vi "CC Observation Queue GUI.vi"() -> ()   [LabVIEW 2024]
uses:
  Subsystems/SS cluster Script Status Queue.ctl
  typedefs/CC cluster Observation.ctl
  CC enum Observation Status.ctl
  Telescope/CC cluster Telescope Offsets.ctl
  typedefs/CC cluster Observation Dither Options.ctl
  typedefs/CC enum Dither Selection.ctl
  Subsystems/SS typedef cluster Instrument Command Queue Data.ctl
  CC cluster Script State.ctl
  CC cluster Observation Settings.ctl
  CC cluster Air Mass Data.ctl
  Logging/CC enum Current Values Action.ctl
  typedefs/CC cluster Script.ctl
  typedefs/CC Script Step.ctl
  typedefs/CC enum Script Action.ctl
  Scripts/CC Rd Wr Script Action.ctl
  hk-channel-class/hk-channel-class/HK Table/HK Table.lvclass
panel:
  in  "Open Plots":bool
  in  "Air Mass Tool":bool
  out "Row":i32 caption="Next"
  in  "queue idle":string="TELESCOPE IDLE"
  in  "clean table":bool
  in  "Auto Step":bool
  in  "Stop":bool
  out "Queue Running":i16(slide) scale=-1.0..70.0
  in  "Pause Q":bool
  in  "Run Queue":bool
  in  "Close":bool
  out "Queue":i32(listbox)
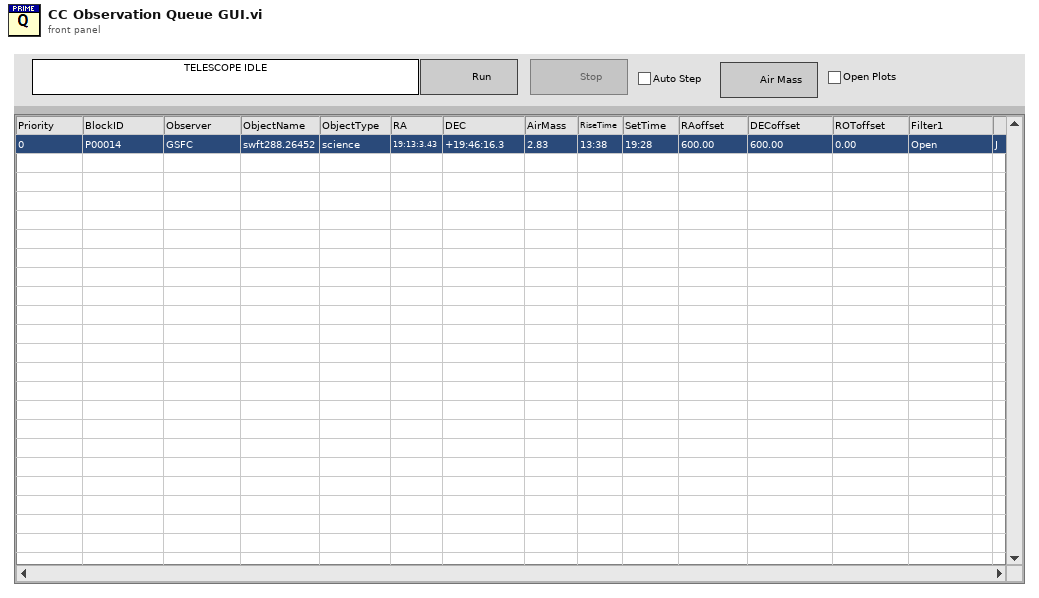
[diagram p1: front panel]
types:
  T1 = typedef "CC cluster Observation.ctl" = cluster{"Priority":i32, "ID":string, "Observer":string, "Obj Name":string, "Obj Type":string, "RA and DEC String":cluster{"RA":string, "DEC":string}, "Filter Wheel 1":string, "Filter Wheel 2":string, "Integration Time":dbl, "Observation Status":T2, "Offsets":T3, "Images":i32, "Dither Options":T4, "Comment 1":string, "Comment 2":string}
  T2 = typedef "CC enum Observation Status.ctl" = enum16{"Ready", "Running", "Done", "Error"}
  T3 = typedef "CC cluster Telescope Offsets.ctl" = cluster{"RA":dbl, "DEC":dbl, "ROT":dbl}
  T4 = typedef "CC cluster Observation Dither Options.ctl" = cluster{"Dither":T5, "Dither Radius":dbl, "Dither Points":i32, "Dither Phase":dbl}
  T5 = typedef "CC enum Dither Selection.ctl" = enum16{"None", "Circle", "Random"}
  T6 = typedef "CC cluster Script State.ctl" = cluster{"Image Count":i32, "Step":i32, "Dither Idx":i32, "Dither Total":i32, "Running":bool, "State":u16}
  T7 = typedef "CC cluster Observation Settings.ctl" = cluster{"Air Mass Program Path":path}
  T8 = typedef "CC cluster Air Mass Data.ctl" = cluster{"BlockID":string, "Air Mass":string, "Rise Time":string, "Set Time":string}
  T9 = cluster{"state":refnum<user-event>, "Obs Queue":refnum<queue>, "Observation List":T1[], "Data":variant, "Obs State":enum16{"Idle", "Running", "Paused"}, "Row":i32, "Script Q":refnum<queue>, "Expected Images":i32, "Script Status":T6, "Prev Status":T6, "script name":string, "Observation Settings":T7, "BlockIDs":string[], "Airmass Idx":i32, "Air Mass":T8[]}
  T10 = typedef "CC enum Current Values Action.ctl" = enum16{"Init", "Write Item", "Write Array", "Read Item", "Read Array", "Read All", "Add Channels", "New File", "Add Message", "Get Current Values", "Close"}
  T11 = enum8{"Enabled", "Disabled", "Disabled and Grayed Out"}
  T12 = typedef "SS typedef cluster Instrument Command Queue Data.ctl" = cluster{"Cmd":string, "Parameters":variant}
  T13 = typedef "CC Rd Wr Script Action.ctl" = enum16{"Read", "Write", "List", "Delete"}
  T14 = typedef "CC cluster Script.ctl" = cluster{"Name":string, "Script":T15[]}
  T15 = typedef "CC Script Step.ctl" = cluster{"Action":T16, "Data":variant}
  T16 = typedef "CC enum Script Action.ctl" = enum16{"Noop", "Define Object", "Define Exposure", "Define Dithering", "Acquire Images", "Set Filter Wheel", "Telescope Home", "Telescope Move", "Telescope RA DEC", "Focus Move Relative", "Focus Move Absolute", "Focus Set Home", "Macro", "Pause", "Ask User", "Define Random Dither"}
  T17 = typedef "SS cluster Script Status Queue.ctl" = cluster{"Msg":string, "Data":variant}
  T18 = typedef "CC cluster Script Panel Defaults.ctl" = cluster{"Script Name":string, "Script Path":path}
  T19 = typedef "LVPoint32TypeDef.ctl" = cluster{"Horizontal":i32, "Vertical":i32}
  T20 = typedef "LVRowAndColumnTypeDef.ctl" = cluster{"Row":i32, "Column":i32}
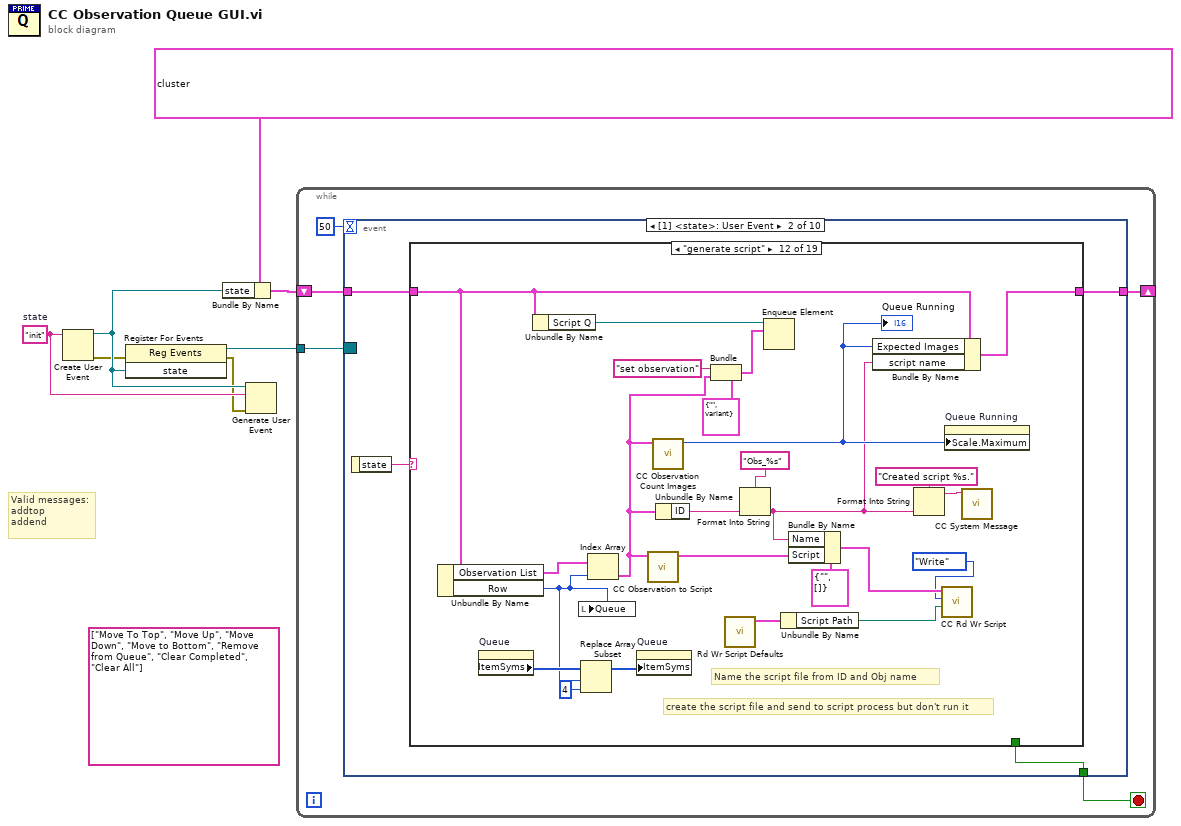
[diagram p0: block diagram]
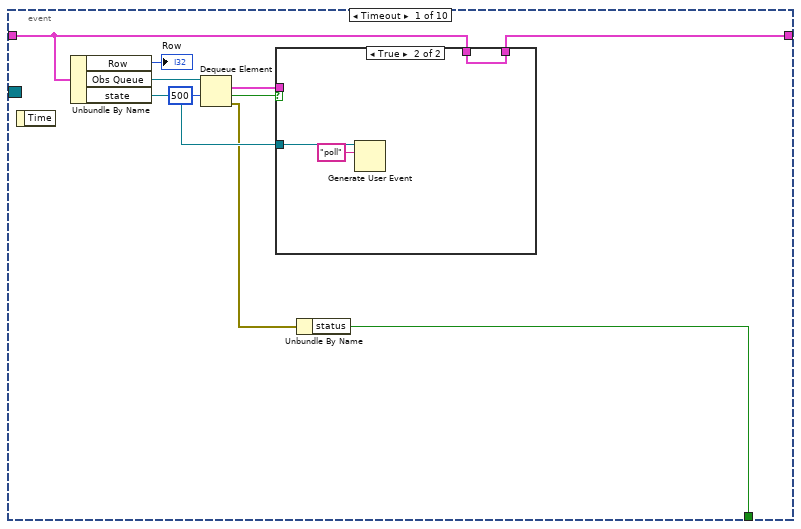
[diagram p2: hidden frame]
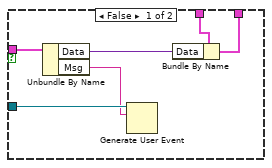
[diagram p3: hidden frame]
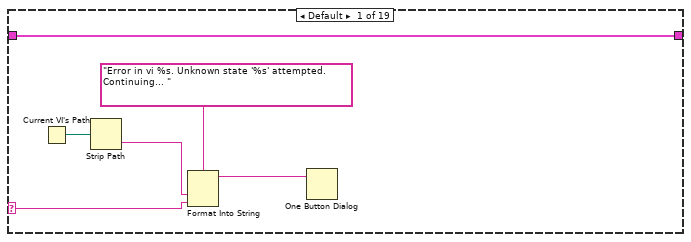
[diagram p4: hidden frame]
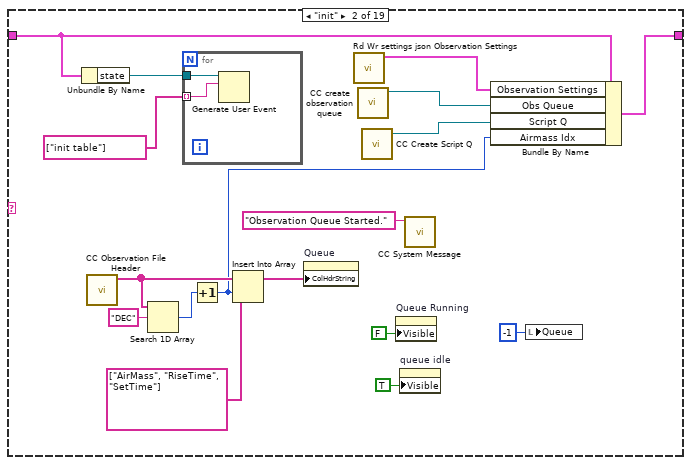
[diagram p5: hidden frame]
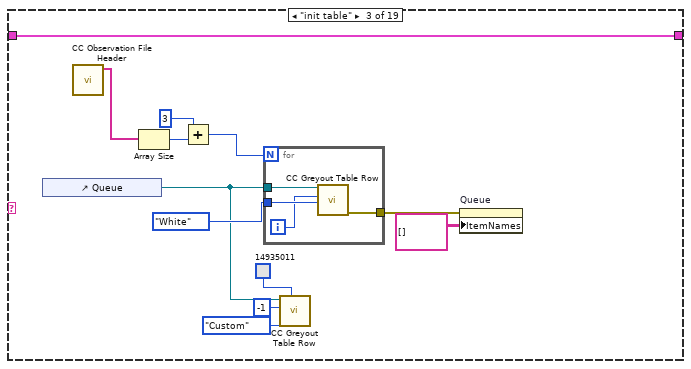
[diagram p6: hidden frame]
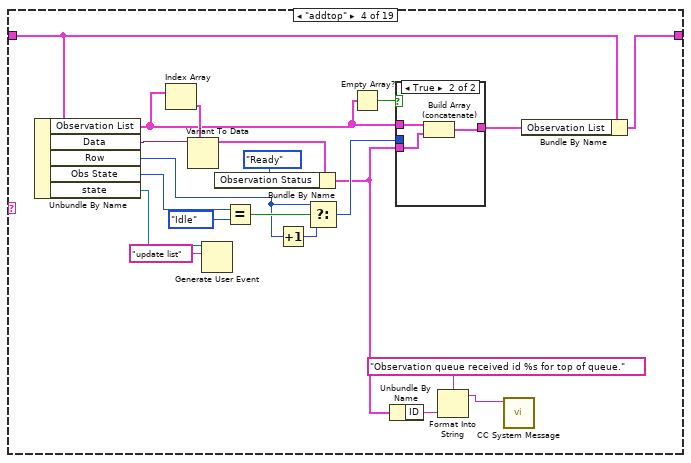
[diagram p7: hidden frame]
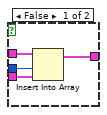
[diagram p8: hidden frame]
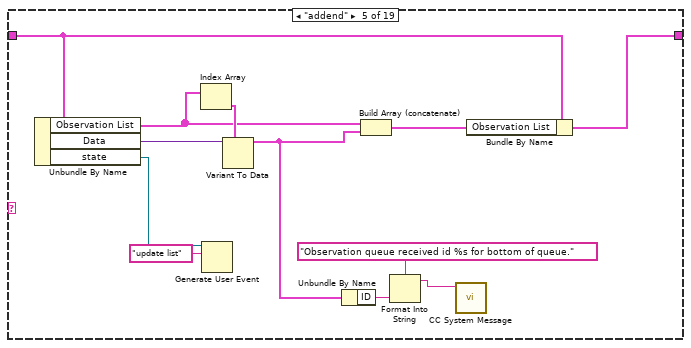
[diagram p9: hidden frame]
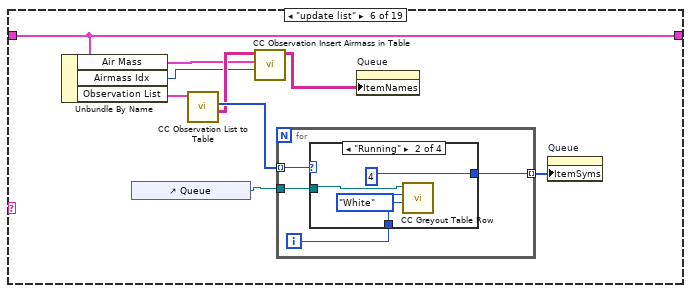
[diagram p10: hidden frame]
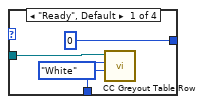
[diagram p11: hidden frame]
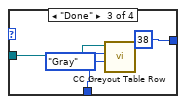
[diagram p12: hidden frame]
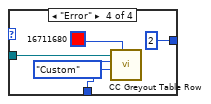
[diagram p13: hidden frame]
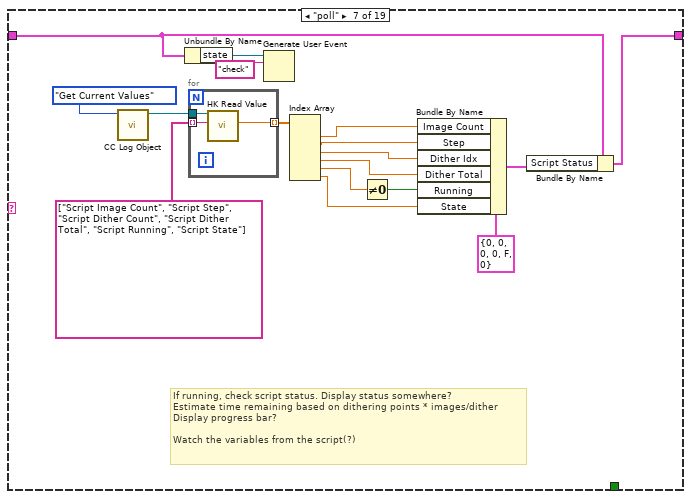
[diagram p14: hidden frame]
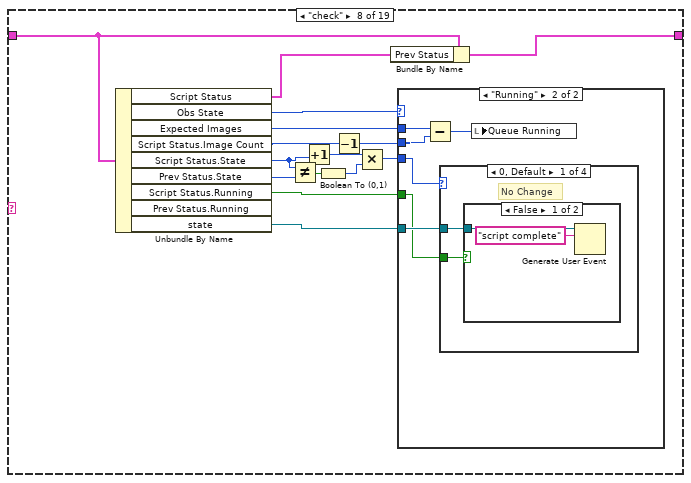
[diagram p15: hidden frame]
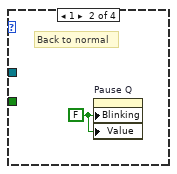
[diagram p18: hidden frame]
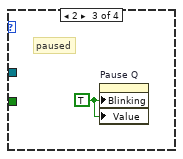
[diagram p19: hidden frame]
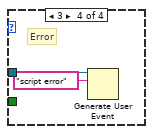
[diagram p20: hidden frame]
diagram:
  (unwired) string[] ["Move To Top", "Move Up", "Move Down", "Move to Bottom", "Remove from Queue", "Clear Completed", "Clear All"]
  w3 = "init"  # state
  # "Valid messages:\naddtop\naddend"
  n1 = Create User Event(user event datatype=w3) -> (user event=w5:refnum<user-event>, error out=w1:errorcluster)  [unwired: 1 in]
  n2 = register-events(error in=w1, w5) -> (reference out=w4:refnum<event-registration>, error out=w2:errorcluster)  [unwired: 1 in]
  n3 = Bundle By Name(cluster=T9 {"state"=refnum, "Obs Queue"=refnum, "Observation List"=[], "Data"=variant, "Obs State"=enum."Idle", "Row"=0, "Script Q"=refnum, "Expected Images"=0, "Script Status"={"Image Count"=0, "Step"=0, "Dither Idx"=0, "Dither Total"=0, "Running"=FALSE, "State"=0}, "Prev Status"={"Image Count"=0, "Step"=0, "Dither Idx"=0, "Dither Total"=0, "Running"=FALSE, "State"=0}, "script name"="", "Observation Settings"={"Air Mass Program Path"=path ""}, "BlockIDs"=["P0102", "P00002", "P00003", "P00004", "P00005", "P00006"], "Airmass Idx"=0, "Air Mass"=[{"BlockID"="", "Air Mass"="", "Rise Time"="06:16", "Set Time"="13:33"}, {"BlockID"="", "Air Mass"="", "Rise Time"="06:16", "Set Time"="13:33"}, {"BlockID"="", "Air Mass"="", "Rise Time"="06:16", "Set Time"="13:33"}, {"BlockID"="", "Air Mass"="", "Rise Time"="06:16", "Set Time"="13:33"}, {"BlockID"="", "Air Mass"="", "Rise Time"="06:16", "Set Time"="13:33"}, {"BlockID"="", "Air Mass"="", "Rise Time"="06:16", "Set Time"="13:33"}]}, "state"=w5) -> (w6:T9)
  n4 = Generate User Event(user event=w5, event data cluster=w3, error in=w2) -> ()  [unwired: 1 in, 2 out]
  n5 = while {
    tunnel: w4 -> [w12]
    shift-right: [w10] -> _
    shift-left: w6 -> [w11]
    stop <- w9 stop-if-true
    n6 = event shown="[1] <state>: User Event" {
      selector: w12 -> [_ _ _ _ _ _ _ _ _ _]
      dyn-events: _ -> [_ _ _ _ _ _ _ _ _ _]
      timeout: 50 -> [_ _ _ _ _ _ _ _ _ _]
      tunnel: w11 -> [w17 w34 w369 w401 w470 w543 w549 w554 w558 w560]
      tunnel: [w18 w33 w370 w401 w471 w543 w549 w554 w558 w560] -> w10
      tunnel: [w14 w32 _ _ _ _ _ _ _ "Close"] -> w9
      event Timeout {
        n7 = event-data() -> ()  [unwired: 1 in, 1 out]
        n8 = Unbundle By Name(w17) -> ("Row"=→"Row":i32, "Obs Queue"=w22:refnum<queue>, "state"=w19:refnum<user-event>)
        n9 = Dequeue Element(queue=w22, timeout in ms (-1)=500) -> (element=w20:T17, timed out?=w21:bool, error out=w15:errorcluster)  [unwired: 1 in, 1 out]
        n10 = case shown="True" w21 {
          tunnel: w20 -> [w28 _]
          tunnel: w19 -> [w27 w30]
          tunnel: w17 -> [w25 w31]
          tunnel: [w23 w31] -> w18
          frame False {
            n11 = Unbundle By Name(w28) -> ("Data"=w24:variant, "Msg"=w26:string)
            n12 = Generate User Event(user event=w27, event data cluster=w26) -> ()  [unwired: 2 in, 2 out]
            n13 = Bundle By Name(cluster=w25, "Data"=w24) -> (w23:T9)
          }
          frame True {
            n14 = Generate User Event(user event=w30, event data cluster="poll" ("event data")) -> ()  [unwired: 2 in, 2 out]
          }
        }
        n15 = Unbundle By Name(w15) -> ("status"=w14:bool)
      }
      event User Event {
        n16 = event-data() -> ("state"=w35:string)  [unwired: 1 in]
        n17 = case shown="\"generate script\"" w35 {
          selector: w35 -> [w40 _ _ _ _ _ _ _ _ _ _ _ _ _ _ _ _ _ _]
          tunnel: w34 -> [w36 w54 w72 w93 w111 w125 w150 w168 w202 w228 w232 w262 w285 w306 w326 w335 w351 w361 w366]
          tunnel: [w36 w57 w72 w94 w112 w125 w151 w169 w203 w229 w233 w273 w286 w307 w326 w336 w352 w361 w366] -> w33
          tunnel: [_ _ _ _ _ _ _ _ _ _ _ _ _ _ _ _ _ _ TRUE] -> w32
          frame Default {
            n18 = Current VI's Path() -> (path=w39:path)
            n19 = Strip Path(path=w39) -> (name=w38:string)  [unwired: 1 out]
            n20 = Format Into String(format string="Error in vi %s. Unknown state '%s' attempted. Continuing... ", w38, w40) -> (resulting string=w37:string)  [unwired: 2 in, 1 out]
            n21 = One Button Dialog(message=w37) -> ()  [unwired: 1 in, 1 out]
          }
          frame "init" {
            n22 = Unbundle By Name(w54) -> ("state"=w53:refnum<user-event>)
            n23 = call "CC Observation File Header.vi"() -> ("Header"=w47:string[])  [unwired: 10 in, 1 out]
            n24 = Search 1D Array(1D array=w47, element="DEC") -> (index of element=w44:i32)  [unwired: 1 in]
            n25 = for {
              tunnel: w53 -> [w60]
              tunnel: string[] ["init table"] -> [w59] mode=indexing
              n26 = Generate User Event(user event=w60, event data cluster=w59) -> ()  [unwired: 2 in, 2 out]
            }
            n27 = Increment(x=w44) -> (x+1=w42:i32)
            n28 = Insert Into Array(array=w47, index=w42, new element=string[] ["AirMass", "RiseTime", "SetTime"]) -> (w45:string[])
            n29 = property on="Queue" class="MCListbox (strict)"("ColHdrString"=w45) -> ()  [unwired: 2 in, 2 out]
            n30 = call "Rd Wr settings json Observation Settings.vi"() -> ("Observation Settings"=w48:T7)  [unwired: 10 in, 1 out]
            n31 = call "CC create observation queue.vi"() -> ("Observation Queue"=w58:refnum<queue>)  [unwired: 10 in, 1 out]
            n32 = call "CC Create Script Q.vi"() -> ("Script Q"=w56:refnum<queue>)  [unwired: 10 in, 1 out]
            n33 = property on="Queue Running" class="Slide (strict)"("Visible"=FALSE) -> ()  [unwired: 2 in, 2 out]
            n34 = property on="queue idle" class="Str"("Visible"=TRUE) -> ()  [unwired: 2 in, 2 out]
            n35 = call "CC System Message.vi"("Message"="Observation Queue Started.") -> ()  [unwired: 10 in, 1 out]
            n36 = Bundle By Name(cluster=w54, "Observation Settings"=w48, "Obs Queue"=w58, "Script Q"=w56, "Airmass Idx"=w42) -> (w57:T9)
            n37 = local write "Queue"(-1 ("Queue")) -> ()
          }
          frame "init table" {
            n38 = control-ref of="Queue"() -> (w68:refnum<vi>)
            n39 = call "CC Observation File Header.vi"() -> ("Header"=w64:string[])  [unwired: 10 in, 1 out]
            n40 = Array Size(array=w64) -> (size(s)=w63:i32)
            n41 = Add(x=3, y=w63) -> (x+y=w62:i32)
            n42 = for {
              N: w62 -> [_]
              tunnel: w68 -> [w76]
              tunnel: [w75] -> w71
              tunnel: enum16{"White", "Gray", "Custom"}."White" ("Color") -> [w74]
              i -> [w73]
              n43 = call "CC Greyout Table Row.vi"("Color"=w74, "Row"=w73, "Queue ref"=w76) -> ("error out"=w75:errorcluster)  [unwired: 8 in]
            }
            n44 = call "CC Greyout Table Row.vi"("Color Box"=u32 14935011, "Color"=enum16{"White", "Gray", "Custom"}."Custom", "Row"=-1, "Queue ref"=w68) -> ()  [unwired: 7 in, 1 out]
            n45 = property on="Queue" class="MCListbox (strict)"(error in=w71, "ItemNames"=string[][] [] ("Item Names")) -> ()  [unwired: 1 in, 2 out]
          }
          frame "addtop" {
            n46 = Unbundle By Name(w93) -> ("Observation List"=w82:T1[], "Data"=w97:variant, "Row"=w77:i32, "Obs State"=w92:enum16{"Idle", "Running", "Paused"}, "state"=w87:refnum<user-event>)
            n47 = Index Array(array=w82) -> (element=w96:T1)  [unwired: 1 in]
            n48 = Variant To Data(type=w96, Variant=w97) -> (data=w81:T1)  [unwired: 1 in, 1 out]
            n49 = Generate User Event(user event=w87, event data cluster="update list" ("event data")) -> ()  [unwired: 2 in, 2 out]
            n50 = Bundle By Name(cluster=w81, "Observation Status"=CC_enum_Observation_Status."Ready") -> (w79:T1)
            n51 = Equal?(x=w92, y=enum16{"Idle", "Running", "Paused"}."Idle") -> (x = y?=w90:bool)
            n52 = Increment(x=w77) -> (x+1=w88:i32)
            n53 = Select(t=w77, s=w90, f=w88) -> (s? t:f=w89:i32)
            n54 = Empty Array?(array=w82) -> (empty?=w78:bool)
            n55 = Unbundle By Name(w79) -> ("ID"=w84:string)
            n56 = case shown="True" w78 {
              tunnel: [w101 w102] -> w95
              tunnel: w89 -> [w100 _]
              tunnel: w82 -> [w99 w104]
              tunnel: w79 -> [w98 w103]
              frame False {
                n57 = Insert Into Array(array=w99, index=w100, new element=w98) -> (w101:T1[])
              }
              frame True {
                n58 = Build Array (concatenate)(w104, w103) -> (w102:T1[])
              }
            }
            n59 = Format Into String(format string="Observation queue received id %s for top of queue.", w84) -> (resulting string=w83:string)  [unwired: 2 in, 1 out]
            n60 = call "CC System Message.vi"("Message"=w83) -> ()  [unwired: 10 in, 1 out]
            n61 = Bundle By Name(cluster=w93, "Observation List"=w95) -> (w94:T9)
          }
          frame "addend" {
            n62 = Unbundle By Name(w111) -> ("Observation List"=w114:T1[], "Data"=w116:variant, "state"=w110:refnum<user-event>)
            n63 = Index Array(array=w114) -> (element=w115:T1)  [unwired: 1 in]
            n64 = Generate User Event(user event=w110, event data cluster="update list" ("event data")) -> ()  [unwired: 2 in, 2 out]
            n65 = Variant To Data(type=w115, Variant=w116) -> (data=w105:T1)  [unwired: 1 in, 1 out]
            n66 = Unbundle By Name(w105) -> ("ID"=w107:string)
            n67 = Build Array (concatenate)(w114, w105) -> (w113:T1[])
            n68 = Format Into String(format string="Observation queue received id %s for bottom of queue.", w107) -> (resulting string=w106:string)  [unwired: 2 in, 1 out]
            n69 = call "CC System Message.vi"("Message"=w106) -> ()  [unwired: 10 in, 1 out]
            n70 = Bundle By Name(cluster=w111, "Observation List"=w113) -> (w112:T9)
          }
          frame "update list" {
            n71 = Unbundle By Name(w125) -> ("Air Mass"=w119:T8[], "Airmass Idx"=w118:i32, "Observation List"=w124:T1[])
            n72 = control-ref of="Queue"() -> (w121:refnum<vi>)
            n73 = call "CC Observation List to Table.vi"("Observation List"=w124) -> ("Screen Ready Table"=w120:string[][], "Status"=w123:T2[])  [unwired: 7 in, 2 out]
            n74 = call "CC Observation Insert Airmass in Table.vi"("Airmass Idx"=w118, "Air Mass"=w119, "Table"=w120) -> ("Table out"=w117:string[][])  [unwired: 8 in]
            n75 = for {
              tunnel: w123 -> [w129] mode=indexing
              tunnel: [w128] -> w122 mode=indexing
              tunnel: w121 -> [w126]
              i -> [w127]
              n76 = case shown="\"Running\"" w129 {
                tunnel: [0 4 ("new element/subarray") 38 ("new element/subarray") 2 ("new element/subarray")] -> w128
                tunnel: w127 -> [w132 w137 w140 w143]
                tunnel: w126 -> [w130 w136 w139 w145]
                frame "Ready", Default {
                  n77 = call "CC Greyout Table Row.vi"("Color"=enum16{"White", "Gray", "Custom"}."White", "Row"=w132, "Queue ref"=w130) -> ()  [unwired: 8 in, 1 out]
                }
                frame "Running" {
                  n78 = call "CC Greyout Table Row.vi"("Color"=enum16{"White", "Gray", "Custom"}."White", "Row"=w137, "Queue ref"=w136) -> ()  [unwired: 8 in, 1 out]
                }
                frame "Done" {
                  n79 = call "CC Greyout Table Row.vi"("Color"=enum16{"White", "Gray", "Custom"}."Gray", "Row"=w140, "Queue ref"=w139) -> ()  [unwired: 8 in, 1 out]
                }
                frame "Error" {
                  n80 = call "CC Greyout Table Row.vi"("Color Box"=u32 16711680, "Color"=enum16{"White", "Gray", "Custom"}."Custom", "Row"=w143, "Queue ref"=w145) -> ()  [unwired: 7 in, 1 out]
                }
              }
            }
            n81 = property on="Queue" class="MCListbox (strict)"("ItemNames"=w117) -> ()  [unwired: 2 in, 2 out]
            n82 = property on="Queue" class="MCListbox (strict)"("ItemSyms"=w122) -> ()  [unwired: 2 in, 2 out]
          }
          frame "poll" {
            # "If running, check script status. Display status somewhere?\nEstimate time remaining based on dithering points * images/dither\nDisplay progress bar?\n\nWatch the variables from the script(?)"
            n83 = call "CC Log Object.vi"("Action"=CC_enum_Current_Values_Action."Get Current Values") -> ("HK Channel out"=w162:refnum<class "HK Table.lvclass">)  [unwired: 8 in, 2 out]
            n84 = Unbundle By Name(w150) -> ("state"=w148:refnum<user-event>)
            n85 = for {
              tunnel: w162 -> [w166]
              tunnel: string[] ["Script Image Count", "Script Step", "Script Dither Count", "Script Dither Total", "Script Running", "Script State"] -> [w165] mode=indexing
              tunnel: [w164] -> w161 mode=indexing
              n86 = call-dynamic "HK Read Value.vi"("Channel Name"=w165, "HK Channel in"=w166) -> ("Value"=w164:dbl)  [unwired: 4 in, 5 out]
            }
            n87 = Generate User Event(user event=w148, event data cluster="check" ("event data")) -> ()  [unwired: 2 in, 2 out]
            n88 = Index Array(array=w161) -> (element #1=w149:dbl, element #2=w158:dbl, element #3=w157:dbl, element #4=w156:dbl, element #5=w155:dbl, element #6=w153:dbl)  [unwired: 6 in]
            n89 = Not Equal To 0?(x=w155) -> (x != 0?=w154:bool)
            n90 = Bundle By Name(cluster=T6 {"Image Count"=0, "Step"=0, "Dither Idx"=0, "Dither Total"=0, "Running"=FALSE, "State"=0}, "Image Count"=w149, "Step"=w158, "Dither Idx"=w157, "Dither Total"=w156, "Running"=w154, "State"=w153) -> (w152:T6)
            n91 = Bundle By Name(cluster=w150, "Script Status"=w152) -> (w151:T9)
          }
          frame "check" {
            n92 = Unbundle By Name(w168) -> ("Script Status"=w170:T6, "Obs State"=w181:enum16{"Idle", "Running", "Paused"}, "Expected Images"=w180:i32, "Script Status.Image Count"=w179:i32, "Script Status.State"=w177:u16, "Prev Status.State"=w178:u16, "Script Status.Running"=w171:bool, "state"=w172:refnum<user-event>)  [unwired: 1 out]
            n93 = Not Equal?(x=w177, y=w178) -> (x != y?=w175:bool)
            n94 = Increment(x=w177) -> (x+1=w176:u16)
            n95 = Boolean To (0,1)(Boolean=w175) -> (0, 1=w173:i16)
            n96 = Decrement(x=w179) -> (x-1=w167:i32)
            n97 = Multiply(x=w176, y=w173) -> (x*y=w174:u16)
            n98 = Bundle By Name(cluster=w168, "Prev Status"=w170) -> (w169:T9)
            n99 = case shown="\"Running\"" w181 {
              tunnel: w180 -> [_ w187]
              tunnel: w167 -> [_ w185]
              tunnel: w174 -> [_ w184]
              tunnel: w172 -> [_ w183]
              tunnel: w171 -> [_ w182]
              frame "Idle", Default {
              }
              frame "Running" {
                n100 = Subtract(x=w187, y=w185) -> (x-y=w186:i32)
                n101 = case shown="0, Default" w184 {
                  tunnel: w183 -> [w189 _ _ w195]
                  tunnel: w182 -> [w188 _ _ _]
                  frame 0, Default {
                    # "No Change"
                    n102 = case shown="False" w188 {
                      tunnel: w189 -> [w190 _]
                      frame False {
                        n103 = Generate User Event(user event=w190, event data cluster="script complete" ("event data")) -> ()  [unwired: 2 in, 2 out]
                      }
                      frame True {
                      }
                    }
                  }
                  frame 1 {
                    w192 = FALSE ("Blinking")
                    # "Back to normal"
                    n104 = property on="Pause Q" class="Bool (strict)"("Blinking"=w192, "Value"=w192) -> ()  [unwired: 2 in, 2 out]
                  }
                  frame 2 {
                    w193 = TRUE ("Blinking")
                    # "paused"
                    n105 = property on="Pause Q" class="Bool (strict)"("Blinking"=w193, "Value"=w193) -> ()  [unwired: 2 in, 2 out]
                  }
                  frame 3 {
                    # "Error"
                    n106 = Generate User Event(user event=w195, event data cluster="script error" ("event data")) -> ()  [unwired: 2 in, 2 out]
                  }
                }
                n107 = local write "Queue Running"(w186) -> ()
              }
            }
          }
          frame "add to top" {
            n108 = Unbundle By Name(w202) -> ("Data"=w209:variant, "Obs State"=w208:enum16{"Idle", "Running", "Paused"}, "Row"=w207:i32, "Observation List"=w206:T1[], "state"=w201:refnum<user-event>)
            n109 = Variant To Data(type=T1 {"Priority"=0, "ID"="", "Observer"="", "Obj Name"="", "Obj Type"="", "RA and DEC String"={"RA"="", "DEC"=""}, "Filter Wheel 1"="", "Filter Wheel 2"="", "Integration Time"=0.0, "Observation Status"=enum."Error", "Offsets"={"RA"=0.0, "DEC"=0.0, "ROT"=0.0}, "Images"=0, "Dither Options"={"Dither"=enum."Random", "Dither Radius"=0.0, "Dither Points"=0, "Dither Phase"=0.0}, "Comment 1"="", "Comment 2"=""} ("Observation"), Variant=w209) -> (data=w205:T1)  [unwired: 1 in, 1 out]
            n110 = Generate User Event(user event=w201, event data cluster="update list" ("event data")) -> ()  [unwired: 2 in, 2 out]
            n111 = case shown="\"Idle\", Default" w208 {
              tunnel: w207 -> [_ w219]
              tunnel: w206 -> [w214 w218]
              tunnel: w205 -> [w211 w215]
              tunnel: [w212 w216] -> w204
              tunnel: [w211 w215] -> w198
              frame "Idle", Default {
                n112 = Insert Into Array(array=w214, index=0, new element=w211) -> (w212:T1[])
              }
              frame "Running", "Paused" {
                n113 = Increment(x=w219) -> (x+1=w217:i32)
                n114 = Insert Into Array(array=w218, index=w217, new element=w215) -> (w216:T1[])
              }
            }
            n115 = Unbundle By Name(w198) -> ("ID"=w197:string)
            n116 = Format Into String(format string="Observation ID %s added to top of Queue" ("Message"), w197) -> (resulting string=w196:string)  [unwired: 2 in, 1 out]
            n117 = Bundle By Name(cluster=w202, "Observation List"=w204) -> (w203:T9)
            n118 = call "CC System Message.vi"("Message"=w196) -> ()  [unwired: 10 in, 1 out]
          }
          frame "add to bottom" {
            n119 = Unbundle By Name(w228) -> ("Data"=w230:variant, "Observation List"=w225:T1[], "state"=w227:refnum<user-event>)
            n120 = Variant To Data(type=T1 {"Priority"=0, "ID"="", "Observer"="", "Obj Name"="", "Obj Type"="", "RA and DEC String"={"RA"="", "DEC"=""}, "Filter Wheel 1"="", "Filter Wheel 2"="", "Integration Time"=0.0, "Observation Status"=enum."Error", "Offsets"={"RA"=0.0, "DEC"=0.0, "ROT"=0.0}, "Images"=0, "Dither Options"={"Dither"=enum."Random", "Dither Radius"=0.0, "Dither Points"=0, "Dither Phase"=0.0}, "Comment 1"="", "Comment 2"=""} ("Observation"), Variant=w230) -> (data=w220:T1)  [unwired: 1 in, 1 out]
            n121 = Generate User Event(user event=w227, event data cluster="update list" ("event data")) -> ()  [unwired: 2 in, 2 out]
            n122 = Build Array (concatenate)(w225, w220) -> (w224:T1[])
            n123 = Unbundle By Name(w220) -> ("ID"=w222:string)
            n124 = Format Into String(format string="Observation ID %s added to end of Queue" ("Message"), w222) -> (resulting string=w221:string)  [unwired: 2 in, 1 out]
            n125 = Bundle By Name(cluster=w228, "Observation List"=w224) -> (w229:T9)
            n126 = call "CC System Message.vi"("Message"=w221) -> ()  [unwired: 10 in, 1 out]
          }
          frame "start queue" {
            w247 = T11."Enabled" ("Disabled")
            n127 = Unbundle By Name(w232) -> ("Observation List"=w237:T1[], "Row"=w235:i32, "state"=w249:refnum<user-event>)
            "Queue" <- w235
            n128 = Index Array(array=w237, index=w235) -> (element=w239:T1)
            n129 = control-ref of="Queue"() -> (w243:refnum<vi>)
            n130 = for {
              tunnel: w249 -> [w252]
              tunnel: string[] ["generate script", "start script"] -> [w251] mode=indexing
              n131 = Generate User Event(user event=w252, event data cluster=w251) -> ()  [unwired: 2 in, 2 out]
            }
            n132 = Bundle By Name(cluster=w239, "Observation Status"=CC_enum_Observation_Status."Running") -> (w236:T1)
            n133 = call "CC Greyout Table Row.vi"("Color"=enum16{"White", "Gray", "Custom"}."White", "Row"=w235, "Queue ref"=w243) -> ()  [unwired: 8 in, 1 out]
            n134 = Unbundle By Name(w239) -> ("ID"=w245:string)
            n135 = Replace Array Subset(array=w237, new element=w236, index=w235) -> (w234:T1[])
            n136 = property on="Pause Q" class="Bool (strict)"("DisabledEnum"=w247) -> ()  [unwired: 2 in, 2 out]
            n137 = Format Into String(format string="Starting Observation %s" ("Message"), w245) -> (resulting string=w244:string)  [unwired: 2 in, 1 out]
            n138 = property on="Stop" class="Bool"("DisabledEnum"=w247) -> ()  [unwired: 2 in, 2 out]
            n139 = Bundle By Name(cluster=w232, "Observation List"=w234) -> (w233:T9)
            n140 = property on="Run Queue" class="Bool"("DisabledEnum"=T11."Disabled and Grayed Out" ("Disabled")) -> ()  [unwired: 2 in, 2 out]
            n141 = call "CC System Message.vi"("Message"=w244) -> ()  [unwired: 10 in, 1 out]
            n142 = property on="Queue Running" class="Slide (strict)"("Visible"=TRUE) -> ()  [unwired: 2 in, 2 out]
            n143 = property on="queue idle" class="Str"("Visible"=FALSE) -> ()  [unwired: 2 in, 2 out]
          }
          frame "generate script" {
            # "Name the script file from ID and Obj name"
            # "create the script file and send to script process but don't run it"
            n144 = Unbundle By Name(w262) -> ("Observation List"=w272:T1[], "Row"=w271:i32)
            n145 = property on="Queue" class="MCListbox (strict)"() -> ("ItemSyms"=w276:i32[])  [unwired: 2 in, 2 out]
            n146 = Unbundle By Name(w262) -> ("Script Q"=w254:refnum<queue>)
            n147 = local write "Queue"(w271) -> ()
            n148 = Replace Array Subset(array=w276, new element=4 ("new element/subarray"), index=w271) -> (w274:i32[])
            n149 = Index Array(array=w272, index=w271) -> (element=w255:T1)
            n150 = property on="Queue" class="MCListbox (strict)"("ItemSyms"=w274) -> ()  [unwired: 2 in, 2 out]
            n151 = call "CC Observation to Script.vi"("Observation"=w255) -> ("Script Steps"=w263:T15[])  [unwired: 9 in, 1 out]
            n152 = call "CC Observation Count Images.vi"("element"=w255) -> ("Total Images"=w259:i32)  [unwired: 9 in, 1 out]
            "Queue Running" <- w259
            n153 = Unbundle By Name(w255) -> ("ID"=w269:string)
            n154 = Bundle(cluster=T12 {"Cmd"="", "Parameters"=variant} ("element"), "Cmd"="set observation", "Parameters"=w255) -> (w256:T12)
            n155 = call "Rd Wr Script Defaults.vi"() -> ("Script Settings"=w267:T18)  [unwired: 10 in, 1 out]
            n156 = Format Into String(format string="Obs_%s", w269) -> (resulting string=w253:string)  [unwired: 2 in, 1 out]
            n157 = Enqueue Element(queue=w254, element=w256) -> ()  [unwired: 2 in, 3 out]
            n158 = Unbundle By Name(w267) -> ("Script Path"=w266:path)
            n159 = Bundle By Name(cluster=T14 {"Name"="", "Script"=[]} ("Script"), "Name"=w253, "Script"=w263) -> (w268:T14)
            n160 = Bundle By Name(cluster=w262, "Expected Images"=w259, "script name"=w253) -> (w273:T9)
            n161 = Format Into String(format string="Created script %s.", w253) -> (resulting string=w260:string)  [unwired: 2 in, 1 out]
            n162 = call "CC Rd Wr Script.vi"("Script Path"=w266, "Action"=CC_Rd_Wr_Script_Action."Write", "Script"=w268) -> ()  [unwired: 3 in, 6 out]
            n163 = property on="Queue Running" class="Slide (strict)"("Scale.Maximum"=w259) -> ()  [unwired: 2 in, 2 out]
            n164 = call "CC System Message.vi"("Message"=w260) -> ()  [unwired: 10 in, 1 out]
          }
          frame "start script" {
            # "Wait for script to initialize variables."
            n165 = Unbundle By Name(w285) -> ("Script Q"=w289:refnum<queue>, "script name"=w281:string)
            n166 = Wait (ms)(milliseconds to wait=u32 2000) -> ()  [unwired: 1 out]
            n167 = Bundle By Name(cluster=T12 {"Cmd"="", "Parameters"=variant} ("element"), "Cmd"="set script", "Parameters"=w281) -> (w280:T12)
            n168 = Enqueue Element(queue=w289, element=w280) -> (queue out=w279:refnum<queue>, error out=w277:errorcluster)  [unwired: 2 in, 1 out]
            n169 = Enqueue Element(queue=w279, element=T12 {"Cmd"="start script", "Parameters"=variant}, error in (no error)=w277) -> ()  [unwired: 1 in, 3 out]
            n170 = call "CC System Message.vi"("Message"="Starting Script.") -> ()  [unwired: 10 in, 1 out]
            n171 = Bundle By Name(cluster=w285, "Obs State"=enum16{"Idle", "Running", "Paused"}."Running") -> (w286:T9)
          }
          frame "script complete" {
            n172 = Unbundle By Name(w306) -> ("Row"=w292:i32, "state"=w305:refnum<user-event>, "Observation List"=w293:T1[])
            n173 = Array Size(array=w293) -> (size(s)=w298:i32)
            n174 = Decrement(x=w298) -> (x-1=w297:i32)
            n175 = call "CC System Message.vi"("Message"="Observation Completed.") -> ()  [unwired: 10 in, 1 out]
            n176 = control-ref of="Queue"() -> (w303:refnum<vi>)
            n177 = Less?(x=w292, y=w297) -> (x < y?=w296:bool)
            n178 = property on="Queue" class="MCListbox (strict)"() -> ("ItemSyms"=w311:i32[])  [unwired: 2 in, 2 out]
            n179 = Index Array(array=w293, index=w292) -> (element=w295:T1)
            n180 = Bundle By Name(cluster=w295, "Observation Status"=CC_enum_Observation_Status."Done") -> (w291:T1)
            n181 = And(x=w296, y="Auto Step") -> (x .and. y?=w299:bool)
            n182 = case shown="False" w299 {
              tunnel: w305 -> [w312 w318]
              tunnel: [enum16{"Idle", "Running", "Paused"}."Idle" ("Obs State") enum16{"Idle", "Running", "Paused"}."Running" ("Obs State")] -> w300
              frame False {
                n183 = Generate User Event(user event=w312, event data cluster="queue idle" ("event data")) -> ()  [unwired: 2 in, 2 out]
              }
              frame True {
                n184 = Generate User Event(user event=w318, event data cluster="start queue" ("event data")) -> ()  [unwired: 2 in, 2 out]
                n185 = local write "Queue"(-1 ("Queue")) -> ()
              }
            }
            n186 = Replace Array Subset(array=w311, new element=38 ("new element/subarray"), index=w292) -> (w309:i32[])
            n187 = Replace Array Subset(array=w293, new element=w291, index=w292) -> (w290:T1[])
            n188 = property on="Queue" class="MCListbox (strict)"("ItemSyms"=w309) -> ()  [unwired: 2 in, 2 out]
            n189 = Increment(x=w292) -> (x+1=w308:i32)
            n190 = call "CC Greyout Table Row.vi"("Color"=enum16{"White", "Gray", "Custom"}."Gray", "Row"=w292, "Queue ref"=w303) -> ()  [unwired: 8 in, 1 out]
            n191 = Bundle By Name(cluster=w306, "Row"=w308, "Obs State"=w300, "Observation List"=w290) -> (w307:T9)
          }
          frame "queue idle" {
            w324 = T11."Disabled and Grayed Out" ("Disabled")
            n192 = property on="Queue Running" class="Slide (strict)"("Visible"=FALSE) -> ()  [unwired: 2 in, 2 out]
            n193 = property on="queue idle" class="Str"("Visible"=TRUE) -> ()  [unwired: 2 in, 2 out]
            n194 = One Button Dialog(message="Queued observations completed. Telescope is now idle.") -> ()  [unwired: 1 in, 1 out]
            n195 = property on="Pause Q" class="Bool (strict)"("DisabledEnum"=w324, "Blinking"=FALSE) -> ()  [unwired: 2 in, 2 out]
            n196 = property on="Stop" class="Bool"("DisabledEnum"=w324) -> ()  [unwired: 2 in, 2 out]
            n197 = local write "Queue"(-1 ("Queue")) -> ()
            n198 = property on="Run Queue" class="Bool"("DisabledEnum"=T11."Enabled" ("Disabled")) -> ()  [unwired: 2 in, 2 out]
          }
          frame "script error" {
            n199 = Unbundle By Name(w335) -> ("state"=w334:refnum<user-event>, "Row"=w331:i32, "Observation List"=w332:T1[])
            n200 = property on="Queue" class="MCListbox (strict)"() -> ("ItemSyms"=w341:i32[])  [unwired: 2 in, 2 out]
            n201 = Replace Array Subset(array=w341, new element=2 ("new element/subarray"), index=w331) -> (w339:i32[])
            n202 = Index Array(array=w332, index=w331) -> (element=w329:T1)
            n203 = Bundle By Name(cluster=w329, "Observation Status"=CC_enum_Observation_Status."Error") -> (w328:T1)
            n204 = call "CC System Message.vi"("Message"="Observation Aborted due to error.") -> ()  [unwired: 10 in, 1 out]
            n205 = property on="Queue" class="MCListbox (strict)"("ItemSyms"=w339) -> ()  [unwired: 2 in, 2 out]
            n206 = Generate User Event(user event=w334, event data cluster="queue idle" ("event data")) -> ()  [unwired: 2 in, 2 out]
            n207 = local write "Auto Step"(FALSE ("Auto")) -> ()
            n208 = Replace Array Subset(array=w332, new element=w328, index=w331) -> (w330:T1[])
            n209 = Bundle By Name(cluster=w335, "Obs State"=enum16{"Idle", "Running", "Paused"}."Idle", "Observation List"=w330) -> (w336:T9)
          }
          frame "script abort" {
            n210 = Unbundle By Name(w351) -> ("state"=w350:refnum<user-event>, "Row"=w345:i32, "Observation List"=w344:T1[])
            n211 = local write "Auto Step"(FALSE ("Auto")) -> ()
            n212 = property on="Queue" class="MCListbox (strict)"() -> ("ItemSyms"=w357:i32[])  [unwired: 2 in, 2 out]
            n213 = Index Array(array=w344, index=w345) -> (element=w348:T1)
            n214 = Bundle By Name(cluster=w348, "Observation Status"=CC_enum_Observation_Status."Ready") -> (w347:T1)
            n215 = Replace Array Subset(array=w357, new element=37 ("new element/subarray"), index=w345) -> (w355:i32[])
            n216 = Generate User Event(user event=w350, event data cluster="queue idle" ("event data")) -> ()  [unwired: 2 in, 2 out]
            n217 = property on="Queue" class="MCListbox (strict)"("ItemSyms"=w355) -> ()  [unwired: 2 in, 2 out]
            n218 = Replace Array Subset(array=w344, new element=w347, index=w345) -> (w343:T1[])
            n219 = call "CC System Message.vi"("Message"="Observation Aborted by user") -> ()  [unwired: 10 in, 1 out]
            n220 = Bundle By Name(cluster=w351, "Obs State"=enum16{"Idle", "Running", "Paused"}."Idle", "Observation List"=w343) -> (w352:T9)
          }
          frame "clean table" {
            n221 = control-ref of="Queue"() -> (w360:refnum<vi>)
            n222 = for {
              N: 50 -> [_]
              tunnel: w360 -> [w364]
              i -> [w363]
              n223 = call "CC Greyout Table Row.vi"("Color"=enum16{"White", "Gray", "Custom"}."White", "Row"=w363, "Queue ref"=w364) -> ()  [unwired: 8 in, 1 out]
            }
          }
          frame "shutdown" {
          }
        }
      }
      event "Air Mass Tool": Value Change {
        n224 = event-data() -> ()  [unwired: 1 in, 6 out]
        n225 = Unbundle By Name(w369) -> ("Observation Settings.Air Mass Program Path"=w371:path, "Observation List"=w368:T1[])
        n226 = Empty String/Path?(string/path=w371) -> (empty?=w374:bool)
        n227 = case shown="True" w374 {
          tunnel: [FALSE ("cancelled") w391] -> w373
          tunnel: [w388 w389] -> w372
          tunnel: w371 -> [w388 _]
          frame False {
          }
          frame True {
            n228 = call "File Dialog"() -> ("selected path"=w389:path, "cancelled"=w391:bool, "error out"=w390:errorcluster)  [unwired: 12 in, 1 out]
            n229 = call <vilib>:"Clear Errors.vi"("error in (no error)"=w390) -> ()  [unwired: 5 in, 2 out]
          }
        }
        n230 = case shown="False" w373 {
          tunnel: w372 -> [w382 _]
          tunnel: w369 -> [w379 w386]
          tunnel: [w385 w386] -> w370
          tunnel: w368 -> [w381 _]
          tunnel: "Open Plots" -> [w375 _]
          frame False {
            n231 = call "CC Launch AirMass Calculator.vi"("Show Plots?"=w375, "Observation List"=w381, "AirMass program"=w382) -> ("Air Mass"=w376:T8[], "BlockIDs"=w380:string[])  [unwired: 6 in, 1 out]
            n232 = Unbundle By Name(w379) -> ("state"=w378:refnum<user-event>)
            n233 = Bundle By Name(cluster=w379, "Observation Settings.Air Mass Program Path"=w382, "BlockIDs"=w380, "Air Mass"=w376) -> (w385:T9)
            n234 = Unbundle By Name(w385) -> ("Observation Settings"=w384:T7)
            n235 = Generate User Event(user event=w378, event data cluster="update list" ("event data")) -> ()  [unwired: 2 in, 2 out]
            n236 = call "Rd Wr settings json Observation Settings.vi"("Write? (F:Read)"=TRUE, "Observation Settings"=w384) -> ()  [unwired: 8 in, 2 out]
          }
          frame True {
          }
        }
      }
      event "Queue": Shortcut Menu Activation? {
        n237 = event-data() -> ("MenuRef"=w400:refnum<k9>, "CtlRef"=w404:refnum<vi>, "Coords"=w403:T19)  [unwired: 1 in, 4 out]
        n238 = Unbundle By Name(w401) -> ("Obs State"=w397:enum16{"Idle", "Running", "Paused"}, "Row"=w398:i32, "Observation List"=w396:T1[])
        n239 = invoke class="MCListbox (strict)" method="Point To Row Column"(reference=w404, "Point"=w403) -> ("CellPosition"=w402:T20)  [unwired: 5 in, 6 out]
        n240 = Array Size(array=w396) -> (size(s)=w395:i32)
        n241 = Unbundle By Name(w402) -> ("Row"=w392:i32)
        n242 = Decrement(x=w395) -> (x-1=w393:i32)
        n243 = Equal?(x=w393, y=w392) -> ()  [unwired: 1 out]
        n244 = for {
          tunnel: w400 -> [w411]
          tunnel: string[] ["Move To Top", "Move Up", "Move Down", "Move to Bottom", "Remove from Queue", "Clear Completed", "Clear All"] -> [w410] mode=indexing
          tunnel: w398 -> [w408]
          tunnel: w392 -> [w407]
          tunnel: w397 -> [w406]
          tunnel: w393 -> [w405]
          n245 = case shown="\"Running\", Default" w406 {
            tunnel: w410 -> [w416 w446]
            tunnel: [w415 w445] -> w409
            tunnel: w408 -> [w414 w444]
            tunnel: w407 -> [w413 w443]
            tunnel: w405 -> [w412 w442]
            frame "Running", Default {
              n246 = case shown="\"Move To Top\"" w416 {
                tunnel: [TRUE w418 w422 w426 w432 w437 TRUE FALSE] -> w415
                tunnel: w414 -> [_ w420 w424 w429 w435 w438 _ _]
                tunnel: w413 -> [_ w419 w423 w428 w434 w439 _ _]
                tunnel: w412 -> [_ _ _ w427 w433 _ _ _]
                frame "False", Default {
                }
                frame "Move To Top" {
                  n247 = Less?(x=w420, y=w419) -> (x < y?=w418:bool)
                }
                frame "Move Up" {
                  n248 = Increment(x=w424) -> (x+1=w421:i32)
                  n249 = Less?(x=w421, y=w423) -> (x < y?=w422:bool)
                }
                frame "Move Down" {
                  n250 = Less?(x=w429, y=w428) -> (x < y?=w430:bool)
                  n251 = Less?(x=w428, y=w427) -> (x < y?=w425:bool)
                  n252 = And(x=w430, y=w425) -> (x .and. y?=w426:bool)
                }
                frame "Move to Bottom" {
                  n253 = Less?(x=w435, y=w434) -> (x < y?=w436:bool)
                  n254 = Less?(x=w434, y=w433) -> (x < y?=w431:bool)
                  n255 = And(x=w436, y=w431) -> (x .and. y?=w432:bool)
                }
                frame "Remove from Queue" {
                  n256 = Not Equal?(x=w438, y=w439) -> (x != y?=w437:bool)
                }
                frame "Clear Completed" {
                }
                frame "Clear All" {
                }
              }
            }
            frame "Idle" {
              n257 = case shown="\"Move To Top\"" w446 {
                tunnel: [TRUE TRUE w450 w452 w458 TRUE TRUE TRUE] -> w445
                tunnel: w444 -> [_ _ w449 w455 w461 _ _ _]
                tunnel: w443 -> [_ _ w451 w454 w460 _ _ _]
                tunnel: w442 -> [_ _ _ w453 w459 _ _ _]
                frame "False", Default {
                }
                frame "Move To Top" {
                }
                frame "Move Up" {
                  n258 = Less?(x=w449, y=w451) -> (x < y?=w450:bool)
                }
                frame "Move Down" {
                  n259 = Less?(x=w455, y=w454) -> (x < y?=w457:bool)
                  n260 = Less?(x=w454, y=w453) -> (x < y?=w456:bool)
                  n261 = And(x=w457, y=w456) -> (x .and. y?=w452:bool)
                }
                frame "Move to Bottom" {
                  n262 = Less?(x=w461, y=w460) -> (x < y?=w463:bool)
                  n263 = Less?(x=w460, y=w459) -> (x < y?=w462:bool)
                  n264 = And(x=w463, y=w462) -> (x .and. y?=w458:bool)
                }
                frame "Remove from Queue" {
                }
                frame "Clear Completed" {
                }
                frame "Clear All" {
                }
              }
            }
          }
          n265 = Set Menu Item Info(7:w410, 9:w409, 11:w411) -> ()  [unwired: 4 in, 2 out]
        }
        n266 = event-data("Discard?"=FALSE) -> ()  [unwired: 1 in, 1 out]
      }
      event "Queue": Shortcut Menu Selection (User) {
        n267 = event-data() -> ("CtlRef"=w482:refnum<vi>, "ItemTag"=w483:string, "Coords"=w481:T19)  [unwired: 1 in, 2 out]
        n268 = Unbundle By Name(w470) -> ("state"=w467:refnum<user-event>, "Observation List"=w479:T1[], "Row"=w475:i32, "Obs State"=w478:enum16{"Idle", "Running", "Paused"})
        n269 = invoke class="MCListbox (strict)" method="Point To Row Column"(reference=w482, "Point"=w481) -> ("CellPosition"=w480:T20)  [unwired: 5 in, 6 out]
        n270 = Equal?(x=w478, y=enum16{"Idle", "Running", "Paused"}."Idle") -> (x = y?=w476:bool)
        n271 = Increment(x=w475) -> (x+1=w474:i32)
        n272 = Generate User Event(user event=w467, event data cluster="update list" ("event data")) -> ()  [unwired: 2 in, 2 out]
        n273 = Select(t=w475, s=w476, f=w474) -> (s? t:f=w473:i32)
        n274 = case shown="\"Remove from Queue\"" w483 {
          tunnel: w480 -> [_ w493 w499 w514 w520 w531 _ _]
          tunnel: w479 -> [w485 w492 w501 w505 w521 w530 w536 _]
          tunnel: w475 -> [w484 w486 w494 w503 w515 w526 w533 _]
          tunnel: w473 -> [_ w488 _ _ _ _ _ _]
          tunnel: [w485 w487 w495 w504 w516 w524 w535 _] -> w472
          tunnel: [w484 w486 w494 w503 w515 w522 w532 0 ("Row")] -> w469
          frame "False", Default {
          }
          frame "Move To Top" {
            n275 = Unbundle By Name(w493) -> ("Row"=w491:i32)
            n276 = Delete From Array(array=w492, index=w491) -> (deleted portion=w489:T1, array with subset deleted=w490:T1[])  [unwired: 1 in]
            n277 = Insert Into Array(array=w490, index=w488, new element=w489) -> (w487:T1[])
          }
          frame "Move Up" {
            n278 = Unbundle By Name(w499) -> ("Row"=w497:i32)
            n279 = Delete From Array(array=w501, index=w497) -> (deleted portion=w498:T1, array with subset deleted=w500:T1[])  [unwired: 1 in]
            n280 = Decrement(x=w497) -> (x-1=w496:i32)
            n281 = Insert Into Array(array=w500, index=w496, new element=w498) -> (w495:T1[])
          }
          frame "Move Down" {
            n282 = Unbundle By Name(w514) -> ("Row"=w508:i32)
            n283 = Array Size(array=w505) -> (size(s)=w510:i32)
            n284 = Index Array(array=w505, index=w508) -> (element=w513:T1)
            n285 = Decrement(x=w510) -> (x-1=w509:i32)
            n286 = Add(x=2, y=w508) -> (x+y=w512:i32)
            n287 = Less Or Equal?(x=w509, y=w508) -> (x <= y?=w507:bool)
            n288 = Insert Into Array(array=w505, index=w512, new element=w513) -> (w511:T1[])
            n289 = Delete From Array(array=w511, index=w508) -> (array with subset deleted=w506:T1[])  [unwired: 1 in, 1 out]
            n290 = Select(t=w505, s=w507, f=w506) -> (s? t:f=w504:T1[])
          }
          frame "Move to Bottom" {
            n291 = Unbundle By Name(w520) -> ("Row"=w519:i32)
            n292 = Delete From Array(array=w521, index=w519) -> (deleted portion=w517:T1, array with subset deleted=w518:T1[])  [unwired: 1 in]
            n293 = Build Array (concatenate)(w518, w517) -> (w516:T1[])
          }
          frame "Remove from Queue" {
            n294 = Unbundle By Name(w531) -> ("Row"=w529:i32)
            n295 = Greater Or Equal?(x=w526, y=w529) -> (x >= y?=w528:bool)
            n296 = Delete From Array(array=w530, index=w529) -> (array with subset deleted=w524:T1[])  [unwired: 1 in, 1 out]
            n297 = Decrement(x=w526) -> (x-1=w527:i32)
            n298 = Select(t=w527, s=w528, f=w526) -> (s? t:f=w525:i32)
            n299 = Max & Min(x=0, y=w525) -> (max(x,y)=w522:i32)  [unwired: 1 out]
            n300 = local write "Queue"(w522) -> ()
          }
          frame "Clear Completed" {
            w532 = 0 ("Row")
            n301 = control-ref of="Queue"() -> (w534:refnum<vi>)
            n302 = Split 1D Array(array=w536, index=w533) -> (second subarray=w535:T1[])  [unwired: 1 out]
            n303 = for {
              N: w533 -> [_]
              tunnel: w534 -> [w539]
              i -> [w538]
              n304 = call "CC Greyout Table Row.vi"("Color"=enum16{"White", "Gray", "Custom"}."White", "Row"=w538, "Queue ref"=w539) -> ()  [unwired: 8 in, 1 out]
            }
            n305 = local write "Queue"(w532) -> ()
          }
          frame "Clear All" {
          }
        }
        n306 = Bundle By Name(cluster=w470, "Observation List"=w472, "Row"=w469) -> (w471:T9)
      }
      event "Run Queue": Value Change {
        n307 = event-data() -> ()  [unwired: 1 in, 1 out]
        n308 = Unbundle By Name(w543) -> ("state"=w542:refnum<user-event>)
        n309 = Generate User Event(user event=w542, event data cluster="start queue" ("event data")) -> ()  [unwired: 2 in, 2 out]
      }
      event "Pause Q": Value Change {
        # "send pause or resume"
        # "Send command to pause after complete of the current step in the script"
        n310 = event-data() -> ()  [unwired: 1 in, 6 out]
        n311 = Unbundle By Name(w549) -> ("Script Q"=w548:refnum<queue>)
        n312 = Select(t=T12 {"Cmd"="pause", "Parameters"=variant} ("element"), s="Pause Q", f=T12 {"Cmd"="resume", "Parameters"=variant} ("element")) -> (s? t:f=w544:T12)
        n313 = Enqueue Element(queue=w548, element=w544) -> ()  [unwired: 2 in, 3 out]
      }
      event "Stop": Value Change {
        # "Send abort script command."
        n314 = event-data() -> ()  [unwired: 1 in, 6 out]
        n315 = Unbundle By Name(w554) -> ("state"=w551:refnum<user-event>, "Script Q"=w553:refnum<queue>)
        n316 = Enqueue Element(queue=w553, element=T12 {"Cmd"="abort script", "Parameters"=variant}) -> ()  [unwired: 2 in, 3 out]
        n317 = local write "Auto Step"(FALSE ("Auto")) -> ()
        n318 = Generate User Event(user event=w551, event data cluster="script abort" ("event data")) -> ()  [unwired: 2 in, 2 out]
      }
      event "clean table": Value Change {
        n319 = event-data() -> ()  [unwired: 1 in, 6 out]
        n320 = Unbundle By Name(w558) -> ("state"=w557:refnum<user-event>)
        n321 = Generate User Event(user event=w557, event data cluster="clean table" ("event data")) -> ()  [unwired: 2 in, 2 out]
      }
      event "Close": Value Change {
        n322 = event-data() -> ()  [unwired: 1 in, 2 out]
      }
    }
  }
